vi "dvp Vi Get Black Level State.vi"(10 "pBlackLevelState":i32, 11 "handle":u32) -> (2 "pBlackLevelState out":i32, 3 "function return":u32(ring))   [LabVIEW 2018, in "LabViewDVPCamera.lvlib"]
doc: "LabviewDvp2Api dvpStatus dvpViGetBlackLevelState(dvpHandle handle, BOOL *pBlackLevelState);"
uses:
  LabViewDVPCamera.lvlib
  LabViewDVPCamera/LabViewDVPCamera.dll
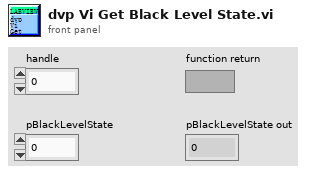
[diagram p1: front panel]
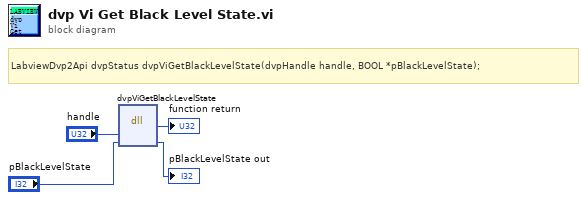
[diagram p0: block diagram]
diagram:
  # "LabviewDvp2Api dvpStatus dvpViGetBlackLevelState(dvpHandle handle, BOOL *pBlackLevelState);"
  n1 = dll-call lib="C:/Program Files (x86)/DVP2 Labview cn 64/Sample/LabViewDVPCamera/LabViewDVPCamera.*" fn="dvpViGetBlackLevelState"("handle"="handle", "pBlackLevelState"="pBlackLevelState") -> (→"function return":u32, "pBlackLevelState"=→"pBlackLevelState out":i32)  [unwired: 4 in, 2 out]
